vi "AssertsSubpanelVI.vi"(11 "error in":errorcluster) -> (15 "error out":errorcluster)   [LabVIEW 2016, in "DronaTest.lvlib"]
uses:
  APIs/Stimulus/ControlValue/SetValueAuto.vi
  APIs/Assert/AssertSubpanel/AssertSubpanelVI.vi
  <vilib>/addons/_JKI Toolkits/Caraya/classes/Assert/Assert Not Error.vi
  <vilib>/addons/_JKI Toolkits/Caraya/classes/Assert/Assert Error.vi
  DronaTest.lvlib
  APIs/Assert/AssertSubpanel/AssertSubpanel.lvlib
  <vilib>/addons/_JKI Toolkits/Caraya/classes/Assert/Assert.lvclass
  Drona.lvlib
  <vilib>/addons/_JKI Toolkits/Caraya/classes/Test/Test.lvclass
  APIs/Stimulus/ControlValue/ControlValue.lvlib
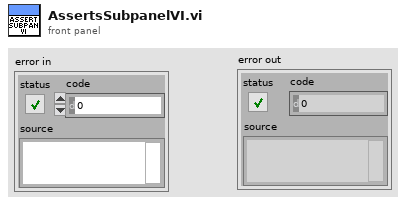
[diagram p1: front panel]
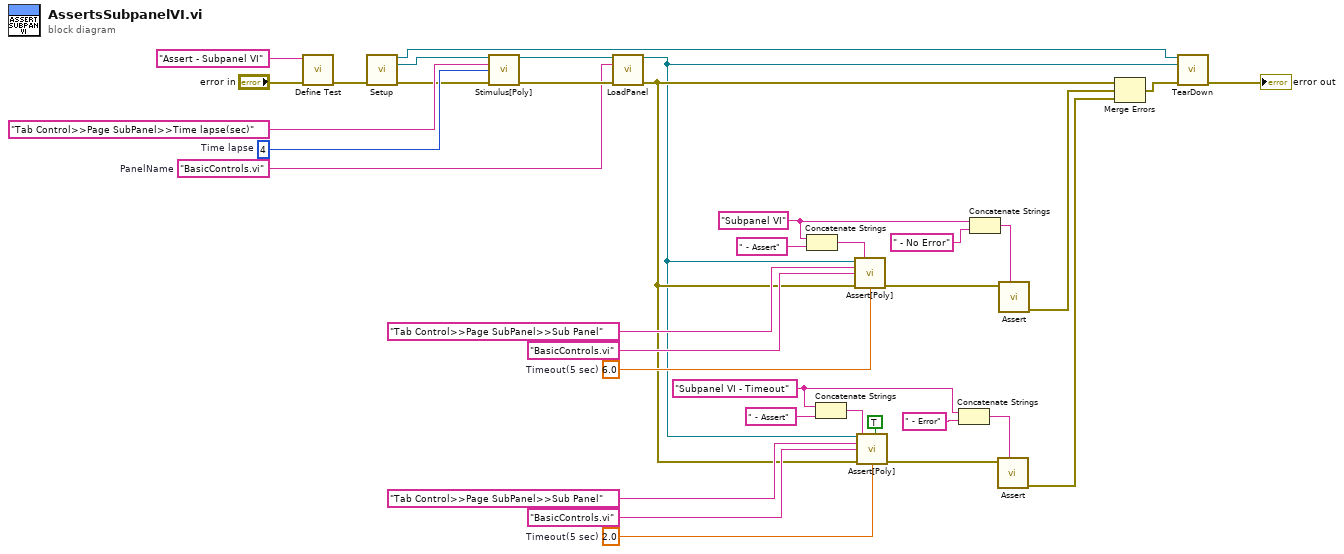
[diagram p0: block diagram]
diagram:
  w21 = "Subpanel VI - Timeout" ("Label")
  w27 = "BasicControls.vi"  # PanelName
  w31 = u32 4  # Time lapse
  w24 = "Subpanel VI" ("Label")
  w17 = 2.0  # Timeout(5 sec)
  w11 = 6.0  # Timeout(5 sec)
  n1 = call <vilib>:"Define Test.vi"("error in (no error)"="error in", "Label (VI Title)"="Assert - Subpanel VI" ("string")) -> ("error out"=w9:errorcluster)  [unwired: 9 in]
  n2 = call "Setup.vi"("error in (no error)"=w9) -> ("Application Ref"=w6:refnum<vi>, "VI out"=w2:refnum<vi>, "error out"=w4:errorcluster)  [unwired: 12 in]
  n3 = call-poly "Stimulus[Poly].vi"("VI Reference In"=w2, "Control Path"="Tab Control>>Page SubPanel>>Time lapse(sec)", "Value (Signaling)"=w31, "error in"=w4) -> ("VI Reference Out"=w29:refnum<vi>, "error out"=w28:errorcluster)  [unwired: 10 in]
  n4 = call "LoadPanel.vi"("VI in"=w29, "Panel Name"=w27, "error in (no error)"=w28) -> ("VI out"=w1:refnum<vi>, "error out"=w3:errorcluster)  [unwired: 11 in]
  n5 = Concatenate Strings(w24, " - Assert" ("string")) -> (w14:string)
  n6 = Concatenate Strings(w21, " - Assert" ("string")) -> (w20:string)
  n7 = call-poly "Assert[Poly].vi"("VI Reference In"=w1, "Test Label"=w14, "Control Path"="Tab Control>>Page SubPanel>>Sub Panel", "VI Name"="BasicControls.vi", "Error In"=w3, "Timeout(5 sec)"=w11) -> ("Error Out"=w10:errorcluster)  [unwired: 8 in, 1 out]
  n8 = call-poly "Assert[Poly].vi"("VI Reference In"=w1, "Test Label"=w20, "Assert Only? (F)"=TRUE, "Control Path"="Tab Control>>Page SubPanel>>Sub Panel", "VI Name"="BasicControls.vi", "Error In"=w3, "Timeout(5 sec)"=w17) -> ("Error Out"=w15:errorcluster)  [unwired: 7 in, 1 out]
  n9 = Concatenate Strings(w21, " - Error" ("string")) -> (w25:string)
  n10 = Concatenate Strings(w24, " - No Error" ("string")) -> (w36:string)
  n11 = call-poly <vilib>:"Assert.vi"("Label"=w25, "Error?"=w15) -> ("error out"=w33:errorcluster)  [unwired: 9 in]
  n12 = call-poly <vilib>:"Assert.vi"("Label"=w36, "Not Error?"=w10) -> ("error out"=w34:errorcluster)  [unwired: 9 in]
  n13 = Merge Errors(w3, w34, w33) -> (w8:errorcluster)
  n14 = call "TearDown.vi"("Application Ref"=w6, "VI in"=w1, "error in (no error)"=w8) -> ("error out"=→"error out":errorcluster)  [unwired: 12 in]
